vi "InputHelper.vi"(3 "error in":errorcluster, 5 "Value":variant) -> (0 "error out":errorcluster, 1 "type":i32, 2 "Wafer ID":string)   [LabVIEW 2012, in "EpiWrapper.lvclass"]
uses:
  EpiWrapper.lvclass
  Controls/UserInput.ctl
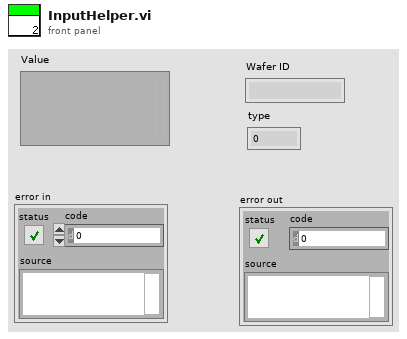
[diagram p1: front panel]
types:
  T1 = typedef "UserInput.ctl" = cluster{"Wafer ID":string, "Test":string, "New":bool, "Save":bool, "Load":bool, "Cancel":bool}
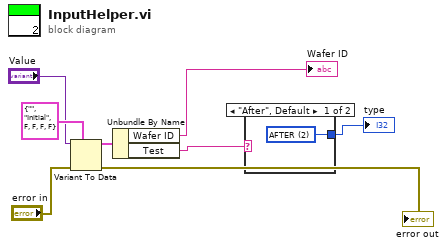
[diagram p0: block diagram]
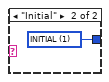
[diagram p2: hidden frame]
diagram:
  n1 = Variant To Data(error in="error in", type=T1 {"Wafer ID"="", "Test"="Initial", "New"=FALSE, "Save"=FALSE, "Load"=FALSE, "Cancel"=FALSE} ("Input"), Variant="Value") -> (data=w5:T1, error out=→"error out":errorcluster)
  n2 = Unbundle By Name(w5) -> ("Wafer ID"=→"Wafer ID":string, "Test"=w6:string)
  n3 = case shown="\"After\", Default" w6 {
    tunnel: [w9 w10] -> w7
    frame "After", Default {
      w9 = 2 items=["INITIAL"=1, "AFTER"=2] ("type")
    }
    frame "Initial" {
      w10 = 1 items=["INITIAL"=1, "AFTER"=2] ("type")
    }
  }
  "type" <- w7
